vi "Has Bits.vi"(8 "error in (no error)":errorcluster, 11 "Packet in":refnum<class "Packet.lvclass">) -> (0 "error out":errorcluster, 2 "Bits Remain":bool, 3 "Packet out":refnum<class "Packet.lvclass">)   [LabVIEW 2020, in "Packet.lvclass"]
uses:
  Packet.lvclass
  Packet.lvclass/Packet.ctl
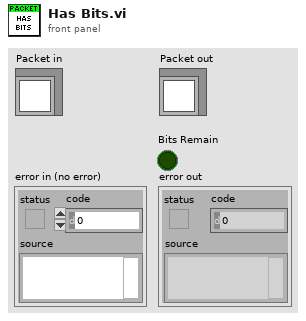
[diagram p1: front panel]
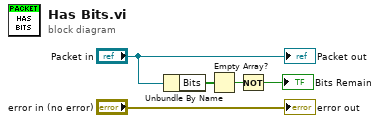
[diagram p0: block diagram]
diagram:
  n1 = Unbundle By Name("Packet in") -> ("Bits"=w3:bool[])
  n2 = Empty Array?(array=w3) -> (empty?=w2:bool)
  n3 = Not(x=w2) -> (.not. x?=→"Bits Remain":bool)
  "error out" <- "error in (no error)"
  "Packet out" <- "Packet in"
